vi "ExecuteSQLQuery.vi"(8 "error in":errorcluster, 10 "SQL query":string, 11 "DB Ref in":T1) -> (0 "error out":errorcluster, 2 "recordset data":variant[][](array[variant]), 3 "DB Ref out":T1, 4 "Data found ?":bool)   [LabVIEW 2013]
uses:
  <vilib>/addons/database/Connection.llb/Conn ObjectReference.ctl
  <vilib>/addons/database/Connection.llb/Conn Execute.vi
  <vilib>/addons/database/Recordset.llb/Rec Fetch Recordset Data (R).vi
  <vilib>/addons/database/Recordset.llb/Rec Destroy - Connection.vi
  <vilib>/addons/database/NI_Database_API.lvlib
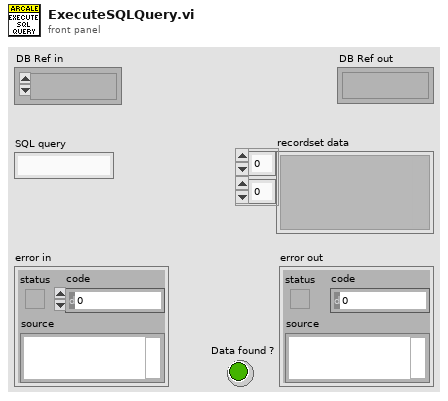
[diagram p1: front panel]
types:
  T1 = typedef "NI_Database_API.lvlib/Conn ObjectReference.ctl" = refnum<k1>
  T2 = typedef "NI_Database_API.lvlib/Rec ObjectReference.ctl" = refnum<k1>
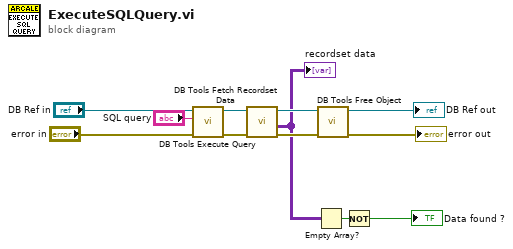
[diagram p0: block diagram]
diagram:
  n1 = call-poly <vilib>:"DB Tools Execute Query.vi"("error in (no error)"="error in", "SQL query"="SQL query", "connection reference"="DB Ref in") -> ("error out"=w8:errorcluster, "recordset reference"=w7:T2)  [unwired: 5 in]
  n2 = call-poly <vilib>:"DB Tools Fetch Recordset Data.vi"("error in (no error)"=w8, "recordset reference"=w7) -> ("error out"=w6:errorcluster, "recordset data"=w2:variant[][], "recordset reference out"=w9:T2)  [unwired: 3 in]
  "recordset data" <- w2
  n3 = Empty Array?(array=w2) -> (empty?=w3:bool)
  n4 = call-poly <vilib>:"DB Tools Free Object.vi"("error in (no error)"=w6, "recordset reference"=w9) -> ("error out"=→"error out":errorcluster, "connection reference"=→"DB Ref out":T1)  [unwired: 8 in]
  n5 = Not(x=w3) -> (.not. x?=→"Data found ?":bool)
